vi "OBD_speed.vi"(11 "COM port":refnum<visa-resource-name>="COM2") -> (3 "Speed (km/h)":u32)   [LabVIEW 2020]
doc: "The Advanced Serial Read and Write example performs a Serial Port Read, a Serial Port Write, or a combination of these actions while setting some advanced serial features like buffer size, termination characters, and XON/XOFF flow control. The user selects the actions (read or write) on the front panel. If both are selected, the VI will write the data first, read the data and then close the VISA session that is opened to the port. \n\nThe parameters set for the serial port must match the parameters of the connected instrument or device. In this example, the bytes to read parameter specifies the number of bytes that the serial port reads. If there were more bytes at the port than the number specified in bytes to read, those bytes would not be read. Also, if you specify to read more bytes than the number of bytes actually read, you might receive a timeout error message.\n\nINSTRUCTIONS:\n1) Select the serial resource and configuration parameters (baud rate, data bits, parity, stop bits, flow control).\n2) Termination character can be enabled and set. Also, set the required input buffer size prior to running the example.\n3) Select the operations to be performed. \n4) Connect the serial port to your device. If no device is available, perform a loopback test by doing one of the following. Short pins 2 and 3 on a RS-232 cable or short pin 4 to pin 8 and pin 5 to pin 9 on a RS-485/422 cable. \n5) Run the VI to see the data read. (The \"read string\" will match the \"string to write\" if a loopback test was performed.)\n\nThis example exposes several advanced features that you may need for your application. Not all applications need all the features shown in this example. The input buffer size is likely an important setting that you want to control in your application. This example expands upon the flow control option for XON and XOFF, allowing the user to choose those control characters. The timeout parameter has been brought to the front panel so a user can specify the time period the VISA Read will wait for the number of bytes to read before timing out. Also, the user has several controls for the termination character, which is discussed later.\n\nNote that you can press the write and read buttons and change the bytes to read parameters on the fly, while the example is running. However, you must stop the example to change the other configuration parameters after the example has started running, and then run again.\n\nSet the I/O buffer size slightly higher the amount of data you expect to receive. This is very important for applications that don't use flow control, as you may lose characters if the receive buffer overflows.\n\nSetting the timeout period ensures that the operation returns with a timeout error if the operation cannot be performed in the specified time period. \n\nSome devices require a termination character in order to identify the end of command strings. Some devices send a termination character to signify the end of data to be read. \n\nThis example shows how you can end the Read operation once a termination character is detected in the buffer and/or append a termination character at the end of the Write data. To enable the Read to end on a termination character, use the VISA Configure Serial Port or use the VISA Properties Serial End Mode for Reads, Termination Character Enable, and Termination Character. To end the Write with a termination character, use the VISA Properties Serial End Mode for Writes, the Send End Enable, and Termination Character. In this example, the same termination character is used for both the Read and the Write. You can specify two different characters for your application, if desired.\n\nYour application may require specific characters for the XON/XOFF Flow Control. You can specify these characters with the VISA Properties Flow Control XOFF Character and Flow Control XON Character. Note that if the standard XON and XOFF characters are used, then decimal 17 and 19 are unavailable for data values. Remember that using flow control and setting an adequate buffer size allow you to prevent buffer overflows."
uses:
  <vilib>/Instr/_visa.llb/VISA Configure Serial Port (Instr).vi
  terminal_test.vi
panel:
  out "Messages":string
  out "Speed (km/h)":u32(graph)
  in  "stop":bool
  in  "?":bool
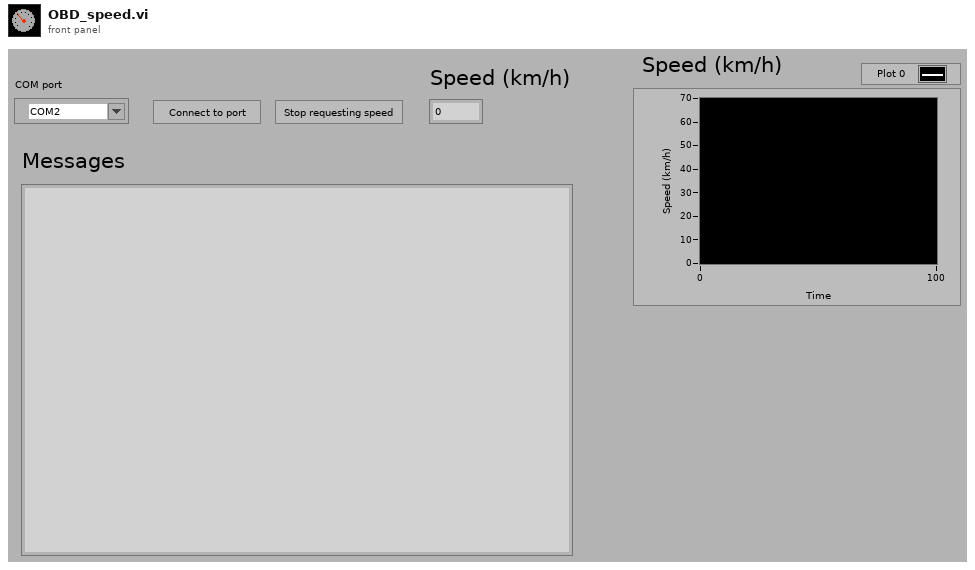
[diagram p1: front panel]
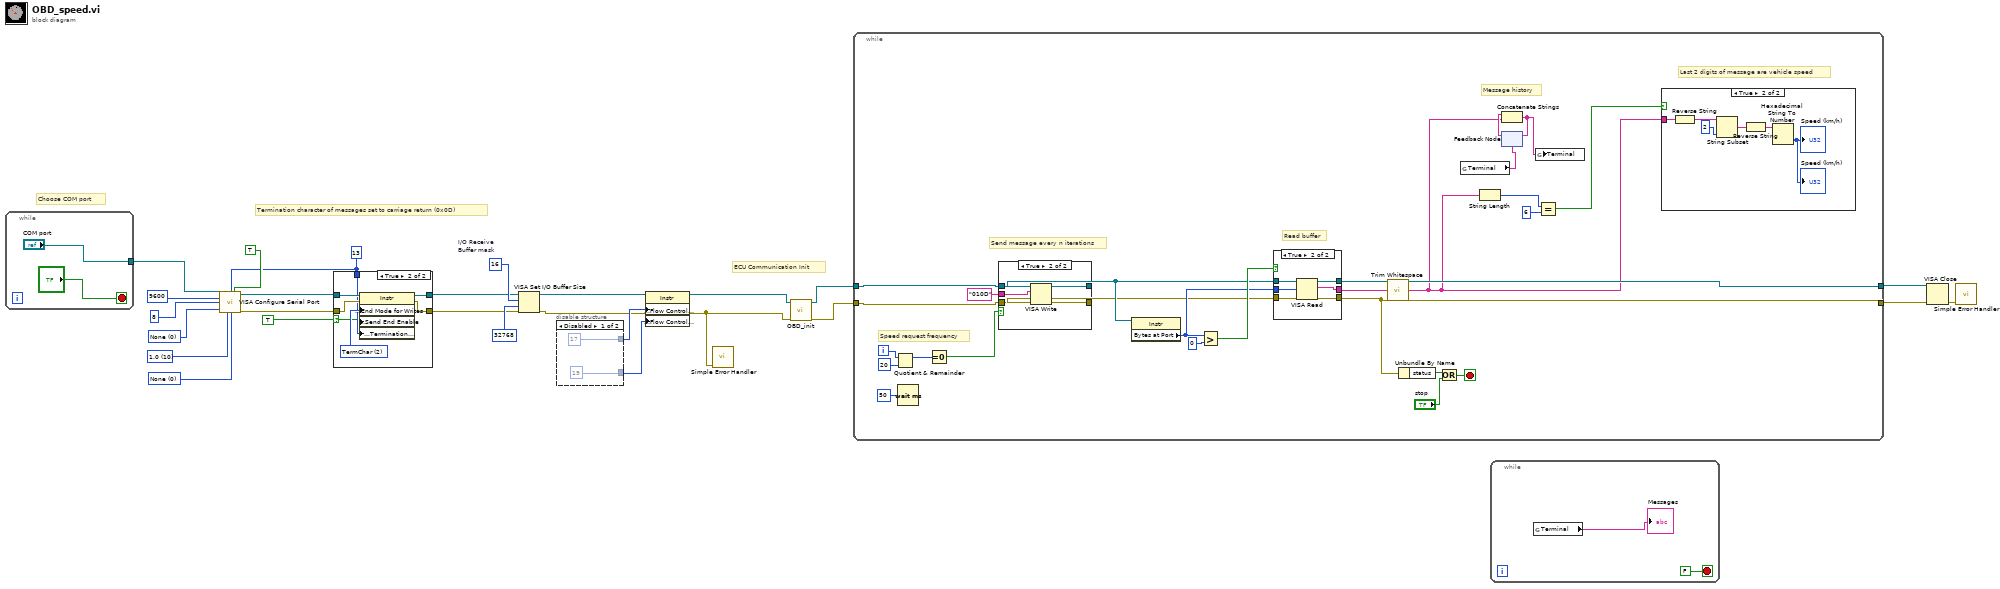
[diagram p0: block diagram]
diagram:
  w18 = u16 0 items=["None"=0, "XON/XOFF"=1, "RTS/CTS"=2, "DTR/DSR"=4] ("flow control")
  w22 = u16 10 items=["1.0"=10, "1.5"=15, "2.0"=20] ("stop bits")
  w12 = u8 13 ("termination char\n(0xA = '\\n' = LF)")
  w23 = u16 0 items=["None", "Odd", "Even", "Mark", "Space"] ("parity")
  w13 = u16 16  # I/O Receive Buffer mask
  # "Termination character of messages set to carriage return (0x0D)"
  # "ECU Communication Init"
  # "Choose COM port"
  n1 = while {
    tunnel: ["COM port"] -> w24
    stop <- "?" stop-if-true
  }
  n2 = call-poly "VISA Configure Serial Port"("VISA resource name"=w24, "termination char\n(0xA = '\\n' = LF)"=w12, "Enable Termination\nChar (T)"=TRUE ("End read on termination character?"), "baud rate (9600)"=u32 9600 ("baud rate"), "data bits (8)"=u16 8 ("data bits"), "parity (0:none)"=w23, "stop bits (10: 1 bit)"=w22, "flow control (0:none)"=w18) -> ("VISA resource name out"=w14:refnum<visa-resource-name>, "error out"=w16:errorcluster)  [unwired: 2 in, 4 out]
  n3 = case shown="True" TRUE ("End write with termination character?") {
    selector: TRUE ("End write with termination character?") -> [_ w30]
    tunnel: w14 -> [w28 w36]
    tunnel: w16 -> [w29 w35]
    tunnel: [w28 w34] -> w7
    tunnel: [w29 w33] -> w15
    tunnel: w12 -> [_ w31]
    frame False {
    }
    frame True {
      w32 = u16 2 items=["None", "LastBit", "TermChar", "Break"] ("Serial Settings:Serial End Mode for Writes")
      n4 = property class="Instr"(reference=w36, error in=w35, "Serial Settings:End Mode for Writes"=w32, "Message Based Settings:Send End Enable"=w30, "Message Based Settings:Termination Character"=w31) -> (reference out=w34:refnum<visa-resource-name>, error out=w33:errorcluster)
    }
  }
  n5 = VISA Set I/O Buffer Size(VISA resource name=w7, mask (16)=w13, size (4096)=u32 32768 ("Input\nbuffer size"), error in (no error)=w15) -> (VISA resource name out=w8:refnum<visa-resource-name>, error out=w4:errorcluster)
  n6 = disable-structure shown="Disabled" {
    disable-tunnel: [u8 17 ("XON Character") _] -> w10
    disable-tunnel: [u8 19 ("XOFF Character") _] -> w9
    frame Disabled {
    }
    frame Enabled {
    }
  }
  n7 = property class="Instr"(reference=w8, "Serial Settings:Flow Control XON Character"=w10, "Serial Settings:Flow Control XOFF Character"=w9) -> (reference out=w3:refnum<visa-resource-name>)  [unwired: 1 in, 1 out]
  n8 = call <vilib>:"Simple Error Handler.vi"("error in (no error)"=w4) -> ()  [unwired: 1 in, 8 out]
  n9 = call "OBD_init.vi"("error in (no error)"=w4, "VISA Refnum in"=w3) -> ("error out"=w1:errorcluster, "VISA Refnum out"=w2:refnum<visa-resource-name>)  [unwired: 8 in]
  n10 = while {
    tunnel: w2 -> [w54]
    tunnel: w1 -> [w53]
    tunnel: [w60] -> w11
    tunnel: [w59] -> w6
    i -> [w49]
    stop <- w43 stop-if-true
    # "Read buffer"
    # "Last 2 digits of message are vehicle speed"
    # "Speed request frequency"
    # "Message history"
    # "Send message every n iterations"
    n11 = Quotient & Remainder(x=w49, y=20) -> (x-y*floor(x/y)=w48:i32)  [unwired: 1 out]
    n12 = Wait (ms)(milliseconds to wait=u32 50) -> ()  [unwired: 1 out]
    n13 = Equal To 0?(x=w48) -> (x = 0?=w47:bool)
    n14 = case shown="True" w47 {
      tunnel: [w80 w85] -> w57
      tunnel: [w79 w84] -> w56
      tunnel: w54 -> [w80 w83]
      tunnel: w53 -> [w79 w82]
      tunnel: "010D" ("String") -> [_ w81]
      frame False {
      }
      frame True {
        n15 = VISA Write(VISA resource name=w83, write buffer=w81, error in (no error)=w82) -> (VISA resource name out=w85:refnum<visa-resource-name>, error out=w84:errorcluster)  [unwired: 1 out]
      }
    }
    n16 = property class="Instr"(reference=w57) -> ("Bytes at Port"=w58:u32)  [unwired: 1 in, 2 out]
    n17 = Greater?(x=w58, y=u32 0) -> (0:w61:bool)
    n18 = case shown="True" w61 {
      tunnel: [w71 w78] -> w59
      tunnel: [w72 w77] -> w60
      tunnel: w56 -> [w71 w76]
      tunnel: w57 -> [w72 w75]
      tunnel: [_ w74] -> w46
      tunnel: w58 -> [_ w73]
      frame False {
      }
      frame True {
        n19 = VISA Read(VISA resource name=w75, byte count=w73, error in (no error)=w76) -> (VISA resource name out=w77:refnum<visa-resource-name>, read buffer=w74:string, error out=w78:errorcluster)  [unwired: 1 out]
      }
    }
    n20 = call <vilib>:"Trim Whitespace.vi"("string"=w46) -> ("trimmed string"=w40:string)  [unwired: 1 in]
    n21 = Unbundle By Name(w59) -> ("status"=w64:bool)
    n22 = Or(x=w64, y="stop") -> (x .or. y?=w43:bool)
    n23 = global read "terminal_test.vi" "Terminal"() -> (w45:string)
    n24 = String Length(string=w40) -> (length=w42:i32)
    n25 = feedback #1(w45) -> (w55:string)
    n26 = Concatenate Strings(w55, w40) -> (w44:string)
    n27 = feedback-in #1(w44) -> ()
    n28 = global write "terminal_test.vi" "Terminal"(w44) -> ()
    n29 = Equal?(x=w42, y=6) -> (x = y?=w39:bool)
    n30 = case shown="True" w39 {
      tunnel: w40 -> [_ w68]
      frame False {
      }
      frame True {
        n31 = Reverse String(1:w68) -> (0:w70:string)
        n32 = String Subset(string=w70, length (rest)=2 ("length (rest)")) -> (substring=w67:string)  [unwired: 1 in]
        n33 = Reverse String(1:w67) -> (0:w66:string)
        n34 = Hexadecimal String To Number(string=w66) -> (number=→"Speed (km/h)" →"Speed (km/h)":u32)  [unwired: 2 in, 1 out]
      }
    }
  }
  n35 = while {
    stop <- FALSE stop-if-true
    n36 = global read "terminal_test.vi" "Terminal"() -> (→"Messages":string)
  }
  n37 = VISA Close(VISA resource name=w11, error in (no error)=w6) -> (error out=w5:errorcluster)
  n38 = call <vilib>:"Simple Error Handler.vi"("error in (no error)"=w5) -> ()  [unwired: 1 in, 8 out]
